vi "PAtestingworks.vi"() -> ()   [LabVIEW 2014]
uses:
  <vilib>/vision/NI_Vision_Development_Module.lvlib
  <instrlib>/KD Scientific 2XX Series/KD Scientific 2XX Series.lvlib
panel:
  in  "Number of Cycles":i32
  in  "Min Pressure":dbl
  in  "Max Pressure":dbl
  out "Status":T1
  in  "stop 2":bool
  out "Delivered Volume":dbl
  out "Units":string
  in  "Baud Rate (9600)":u32(ring)=9600 items=["300"=300, "1200"=1200, "2400"=2400, "4800"=4800, "9600"=9600]
  in  "Withdrawal Settings":T2={"Flow Rate (5)"=5.0, "Volume (10)"=10.0, "Volume Units (ml)"=enum."milliliters (ml)", "Rate Units (ml/min.)"=enum."milliliters per minute (ml/min.)"} {"Volume (10)" format="%#.3g"}
  in  "Diameter (8.75 mm)":dbl=8.75
  in  "Infusion Settings":T2={"Flow Rate (5)"=5.0, "Volume (10)"=10.0, "Volume Units (ml)"=enum."milliliters (ml)", "Rate Units (ml/min.)"=enum."milliliters per minute (ml/min.)"}
  in  "Address (0)":i32 format="%0.0f"
  in  "error in (no error)":errorcluster
  in  "VISA resource name":refnum<visa-resource-name>="COM1"
  in  "stop":bool
  out "Image":T3(plugin-control)
  out "Particle Measurements (Pixels) (Particle Analysis 1)":dbl[][](array[numeric]) format="%.2f"
  out "subarray":dbl[](array[numeric])
  out "The diameter":dbl[](array[numeric])
  in  "stop (F)":bool
  out "Data from Transducer":dynamicdata(graph) caption="Voltage from Transducer V"
  out "Voltage from pressure transducer":dbl[](array[numeric])
  out "Pressure mm Hg":dbl[](graph)
  in  "Calibration factor":dbl[](array[numeric])
  in  "Zero Error":dbl[](array[numeric])
  out "pressure mm Hg":dbl[](array[numeric])
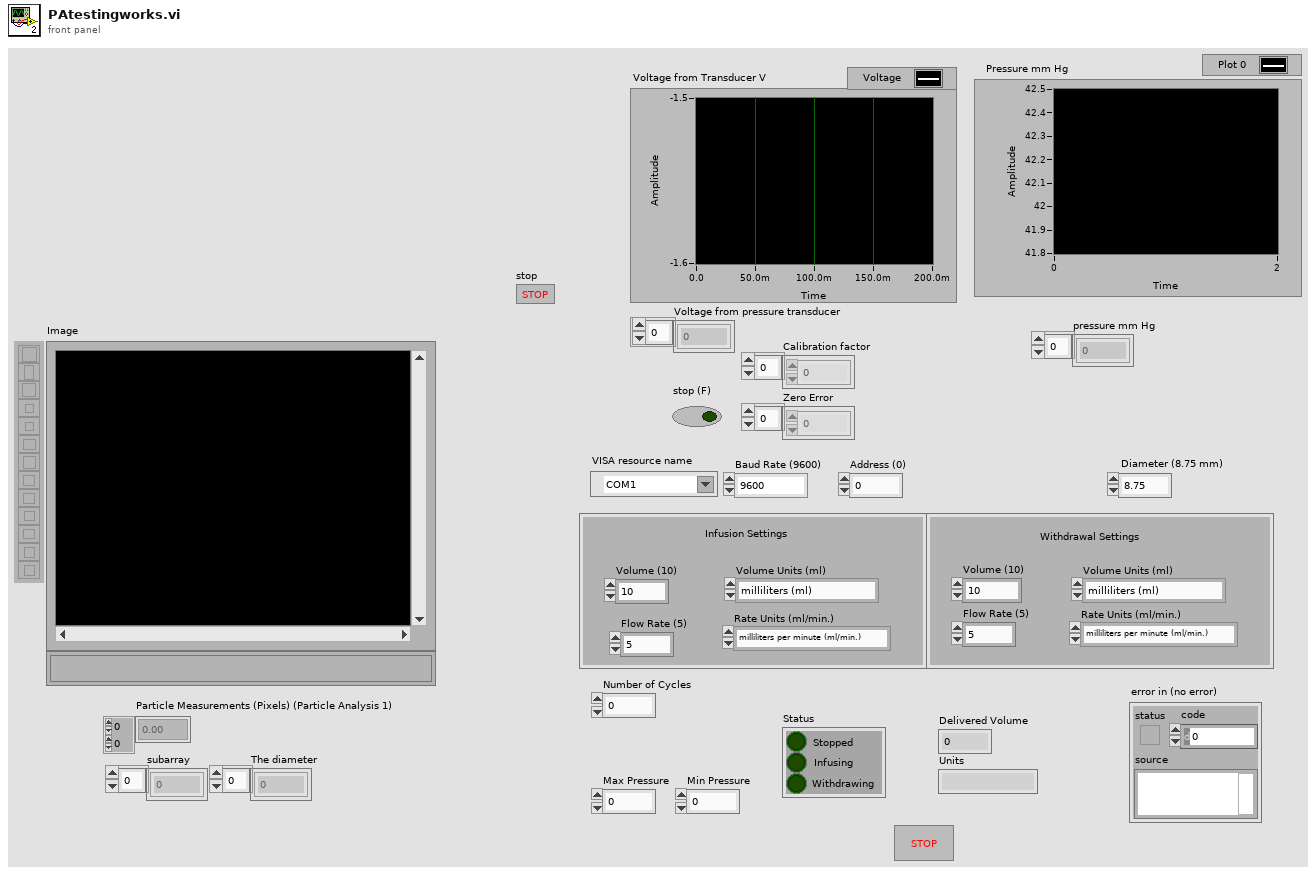
[diagram p1: front panel]
types:
  T1 = cluster{"Stopped":bool, "Infusing":bool, "Withdrawing":bool}
  T2 = cluster{"Flow Rate (5)":dbl, "Volume (10)":dbl, "Volume Units (ml)":enum16{"milliliters (ml)", "microliters (ul)"}, "Rate Units (ml/min.)":enum16{"milliliters per minute (ml/min.)", "milliliters per hour (ml/hr.)", "microliters per minute (ul/min.)", "microliters per hour (ul/hr.)"}}
  T3 = typedef "IMAQ Image.ctl" = refnum<image>
  T4 = typedef "Board Id" = u8
  T5 = typedef "ROI Descriptor" = cluster{"Global Rectangle":i32[], "Contours":cluster{"ID":enum32{"External", "Internal"}, "Type":u32, "Coordinates":i32[]}[]}
  T6 = enum16{"milliliters per minute (ml/min.)", "milliliters per hour (ml/hr.)", "microliters per minute (ul/min.)", "microliters per hour (ul/hr.)"}
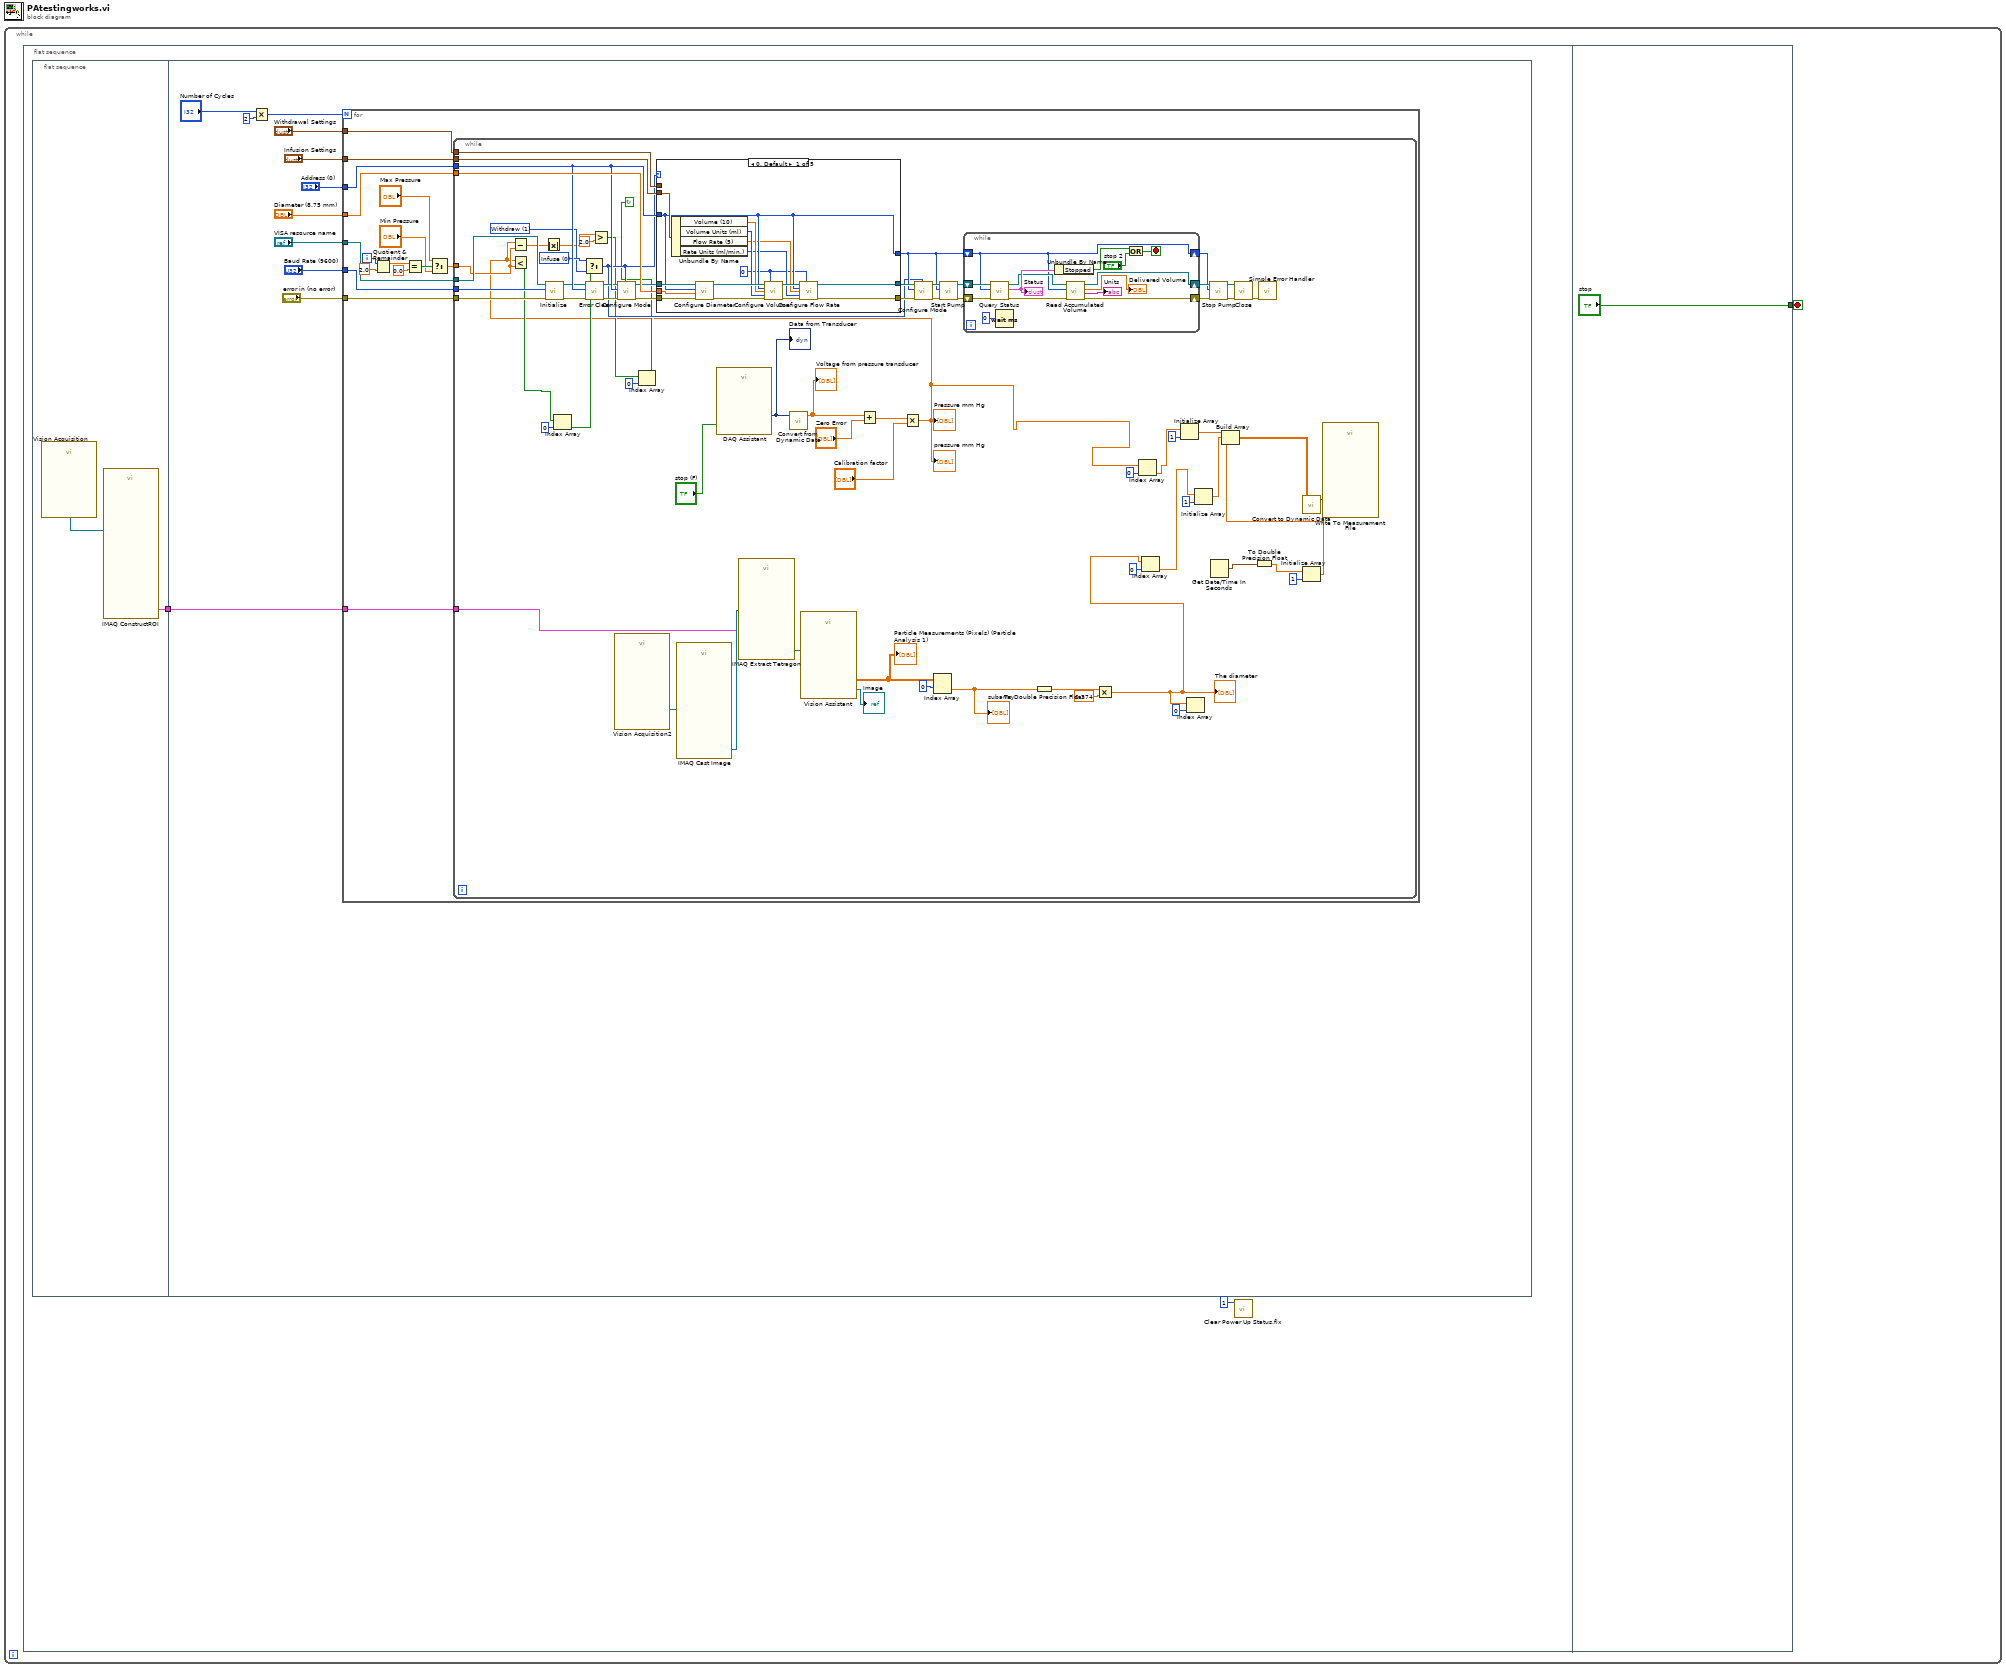
[diagram p0: block diagram]
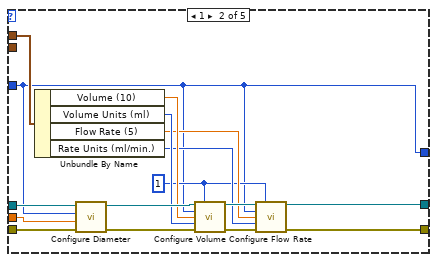
[diagram p2: hidden frame]
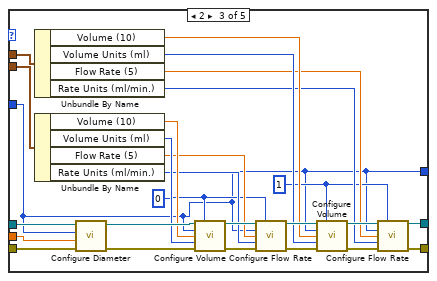
[diagram p3: hidden frame]
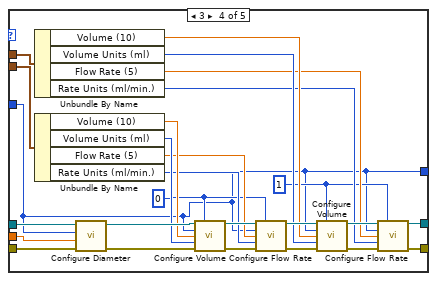
[diagram p4: hidden frame]
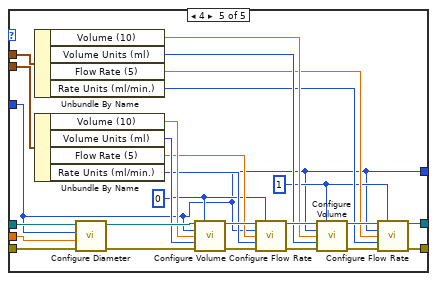
[diagram p5: hidden frame]
diagram:
  n1 = while {
    stop <- w1 stop-if-true
    n2 = flat-sequence {
      tunnel: ["stop"] -> w1
      frame #0 {
        n3 = flat-sequence {
          tunnel: [w4] -> w3
          tunnel: w3 -> [w7]
          frame #0 {
            n4 = call "Vision Acquisition"() -> ("Image Out"=w5:T3)  [unwired: 26 in, 1 out]
            n5 = call "IMAQ ConstructROI"("Image"=w5) -> ("ROI Descriptor Out"=w4:T5)  [unwired: 7 in, 3 out]
          }
          frame #1 {
            n6 = Multiply(x="Number of Cycles", y=2) -> (x*y=w6:i32)
            n7 = for {
              N: w6 -> [_]
              tunnel: "VISA resource name" -> [w32]
              tunnel: "error in (no error)" -> [w31]
              tunnel: "Infusion Settings" -> [w30]
              tunnel: "Withdrawal Settings" -> [w29]
              tunnel: "Diameter (8.75 mm)" -> [w28]
              tunnel: "Baud Rate (9600)" -> [w27]
              tunnel: "Address (0)" -> [w26]
              tunnel: w7 -> [w17]
              i -> [w24]
              n8 = Quotient & Remainder(x=w24, y=2.0) -> (x-y*floor(x/y)=w22:dbl)  [unwired: 1 out]
              n9 = Equal?(x=w22, y=0.0) -> (x = y?=w21:bool)
              n10 = Select(t="Max Pressure", s=w21, f="Min Pressure") -> (s? t:f=w18:dbl)
              n11 = while {
                tunnel: w32 -> [w104]
                tunnel: w31 -> [w103]
                tunnel: w30 -> [w102]
                tunnel: w29 -> [w101]
                tunnel: w28 -> [w100]
                tunnel: w27 -> [w99]
                tunnel: w26 -> [w98]
                tunnel: w18 -> [w75]
                tunnel: w17 -> [w49]
                stop <- w60 continue-if-true
                w77 = u16 1 items=["Withdraw"=1]
                w78 = u16 0 items=["Infuse"] ("Mode (infuse)")
                n12 = call <instrlib>:"Initialize.vi"("error in (no error)"=w103, "Baud Rate (9600)"=w99, "VISA resource name"=w104) -> ("error out"=w80:errorcluster, "VISA resource name out"=w79:refnum<visa-resource-name>)  [unwired: 7 in]
                n13 = call <instrlib>:"Error Clear.vi"("error in (no error)"=w80, "Address (0)"=w98, "VISA resource name"=w79) -> ("error out"=w81:errorcluster, "VISA resource name out"=w82:refnum<visa-resource-name>)  [unwired: 6 in, 1 out]
                n14 = call "Vision Acquisition2"() -> ("Image Out"=w59:T3)  [unwired: 25 in, 2 out]
                n15 = call "IMAQ Cast Image"("Image Src"=w59) -> ("Image Dst Out"=w52:T3)  [unwired: 9 in, 1 out]
                n16 = call "DAQ Assistant"("stop (T)"="stop (F)") -> ("data"=w66:dynamicdata)  [unwired: 16 in, 2 out]
                "Data from Transducer" <- w66
                n17 = call-poly "IMAQ Extract Tetragon"("ROI Descriptor"=w49, "Image Src"=w52) -> ("Image Dst Out"=w51:T3)  [unwired: 8 in, 1 out]
                n18 = call "Convert from Dynamic Data"("Dynamic Data Type"=w66) -> ("Array"=w69:dbl[])  [unwired: 3 in]
                "Voltage from pressure transducer" <- w69
                n19 = call "Vision Assistant"("Image In"=w51) -> ("Image Out"=→"Image":T3, "Particle Measurements (Pixels) (Particle Analysis 1)"=w53:dbl[][])  [unwired: 23 in, 2 out]
                "Particle Measurements (Pixels) (Particle Analysis 1)" <- w53
                n20 = Add(x=w69, y="Zero Error") -> (x+y=w67:dbl[])
                n21 = Multiply(x=w67, y="Calibration factor") -> (x*y=w45:dbl[])
                "Pressure mm Hg" <- w45
                "pressure mm Hg" <- w45
                n22 = Subtract(x=w45, y=w75) -> (x-y=w74:dbl[])
                n23 = Less?(x=w45, y=w75) -> (x < y?=w65:bool[])
                n24 = Absolute Value(x=w74) -> (abs(x)=w73:dbl[])
                n25 = Index Array(array=w65, index=0) -> (element=w63:bool)
                n26 = Select(t=w78, s=w63, f=w77) -> (s? t:f=w76:u16)
                n27 = Greater?(x=w73, y=2.0) -> (0:w62:bool[])
                n28 = call <instrlib>:"Configure Mode.vi"("Mode (infuse)"=w76, "error in (no error)"=w81, "Address (0)"=w98, "VISA resource name"=w82) -> ("error out"=w84:errorcluster, "VISA resource name out"=w83:refnum<visa-resource-name>)  [unwired: 6 in]
                n29 = Index Array(array=w62, index=0) -> (element=w60:bool)
                n30 = case shown="0, Default" w76 {
                  tunnel: w102 -> [w114 _ w162 w188 w214]
                  tunnel: w101 -> [_ w136 w161 w187 w213]
                  tunnel: w83 -> [w120 w135 w160 w186 w212]
                  tunnel: w84 -> [w119 w131 w159 w185 w211]
                  tunnel: w100 -> [w113 w127 w142 w168 w194]
                  tunnel: [w112 w121 w137 w163 w189] -> w85
                  tunnel: w98 -> [w112 w121 w137 w163 w189]
                  tunnel: [w107 w132 w139 w165 w191] -> w89
                  tunnel: [w106 w128 w138 w164 w190] -> w88
                  frame 0, Default {
                    w105 = 0
                    n31 = Unbundle By Name(w114) -> ("Volume (10)"=w111:dbl, "Volume Units (ml)"=w110:enum16{"milliliters (ml)", "microliters (ul)"}, "Flow Rate (5)"=w109:dbl, "Rate Units (ml/min.)"=w108:T6)
                    n32 = call <instrlib>:"Configure Diameter.vi"("error in (no error)"=w119, "Diameter (8.75 mm)"=w113, "Address (0)"=w112, "VISA resource name"=w120) -> ("error out"=w117:errorcluster, "VISA resource name out"=w118:refnum<visa-resource-name>)  [unwired: 6 in]
                    n33 = call <instrlib>:"Configure Volume.vi"("VISA resource name"=w118, "Mode (infuse)"=w105, "Address (0)"=w112, "Volume (100)"=w111, "Units (0: milliliters)"=w110, "error in (no error)"=w117) -> ("VISA resource name out"=w116:refnum<visa-resource-name>, "error out"=w115:errorcluster)  [unwired: 8 in]
                    n34 = call <instrlib>:"Configure Flow Rate.vi"("VISA resource name"=w116, "Mode (infuse)"=w105, "Address (0)"=w112, "Flow Rate (5)"=w109, "Units (0: milliliters per minute)"=w108, "error in (no error)"=w115) -> ("VISA resource name out"=w107:refnum<visa-resource-name>, "error out"=w106:errorcluster)  [unwired: 8 in]
                  }
                  frame 1 {
                    w122 = 1
                    n35 = Unbundle By Name(w136) -> ("Volume (10)"=w126:dbl, "Volume Units (ml)"=w125:enum16{"milliliters (ml)", "microliters (ul)"}, "Flow Rate (5)"=w124:dbl, "Rate Units (ml/min.)"=w123:T6)
                    n36 = call <instrlib>:"Configure Diameter.vi"("error in (no error)"=w131, "Diameter (8.75 mm)"=w127, "Address (0)"=w121, "VISA resource name"=w135) -> ("error out"=w130:errorcluster, "VISA resource name out"=w134:refnum<visa-resource-name>)  [unwired: 6 in]
                    n37 = call <instrlib>:"Configure Volume.vi"("VISA resource name"=w134, "Mode (infuse)"=w122, "Address (0)"=w121, "Volume (100)"=w126, "Units (0: milliliters)"=w125, "error in (no error)"=w130) -> ("VISA resource name out"=w133:refnum<visa-resource-name>, "error out"=w129:errorcluster)  [unwired: 8 in]
                    n38 = call <instrlib>:"Configure Flow Rate.vi"("VISA resource name"=w133, "Mode (infuse)"=w122, "Address (0)"=w121, "Flow Rate (5)"=w124, "Units (0: milliliters per minute)"=w123, "error in (no error)"=w129) -> ("VISA resource name out"=w132:refnum<visa-resource-name>, "error out"=w128:errorcluster)  [unwired: 8 in]
                  }
                  frame 2 {
                    w140 = 1
                    w141 = 0
                    n39 = Unbundle By Name(w161) -> ("Volume (10)"=w146:dbl, "Volume Units (ml)"=w145:enum16{"milliliters (ml)", "microliters (ul)"}, "Flow Rate (5)"=w144:dbl, "Rate Units (ml/min.)"=w143:T6)
                    n40 = Unbundle By Name(w162) -> ("Volume (10)"=w150:dbl, "Volume Units (ml)"=w149:enum16{"milliliters (ml)", "microliters (ul)"}, "Flow Rate (5)"=w148:dbl, "Rate Units (ml/min.)"=w147:T6)
                    n41 = call <instrlib>:"Configure Diameter.vi"("error in (no error)"=w159, "Diameter (8.75 mm)"=w142, "Address (0)"=w137, "VISA resource name"=w160) -> ("error out"=w154:errorcluster, "VISA resource name out"=w158:refnum<visa-resource-name>)  [unwired: 6 in]
                    n42 = call <instrlib>:"Configure Volume.vi"("VISA resource name"=w158, "Mode (infuse)"=w141, "Address (0)"=w137, "Volume (100)"=w150, "Units (0: milliliters)"=w149, "error in (no error)"=w154) -> ("VISA resource name out"=w157:refnum<visa-resource-name>, "error out"=w153:errorcluster)  [unwired: 8 in]
                    n43 = call <instrlib>:"Configure Flow Rate.vi"("VISA resource name"=w157, "Mode (infuse)"=w141, "Address (0)"=w137, "Flow Rate (5)"=w148, "Units (0: milliliters per minute)"=w147, "error in (no error)"=w153) -> ("VISA resource name out"=w156:refnum<visa-resource-name>, "error out"=w152:errorcluster)  [unwired: 8 in]
                    n44 = call <instrlib>:"Configure Volume.vi"("VISA resource name"=w156, "Mode (infuse)"=w140, "Address (0)"=w137, "Volume (100)"=w146, "Units (0: milliliters)"=w145, "error in (no error)"=w152) -> ("VISA resource name out"=w155:refnum<visa-resource-name>, "error out"=w151:errorcluster)  [unwired: 8 in]
                    n45 = call <instrlib>:"Configure Flow Rate.vi"("VISA resource name"=w155, "Mode (infuse)"=w140, "Address (0)"=w137, "Flow Rate (5)"=w144, "Units (0: milliliters per minute)"=w143, "error in (no error)"=w151) -> ("VISA resource name out"=w139:refnum<visa-resource-name>, "error out"=w138:errorcluster)  [unwired: 8 in]
                  }
                  frame 3 {
                    w166 = 1
                    w167 = 0
                    n46 = Unbundle By Name(w187) -> ("Volume (10)"=w172:dbl, "Volume Units (ml)"=w171:enum16{"milliliters (ml)", "microliters (ul)"}, "Flow Rate (5)"=w170:dbl, "Rate Units (ml/min.)"=w169:T6)
                    n47 = Unbundle By Name(w188) -> ("Volume (10)"=w176:dbl, "Volume Units (ml)"=w175:enum16{"milliliters (ml)", "microliters (ul)"}, "Flow Rate (5)"=w174:dbl, "Rate Units (ml/min.)"=w173:T6)
                    n48 = call <instrlib>:"Configure Diameter.vi"("error in (no error)"=w185, "Diameter (8.75 mm)"=w168, "Address (0)"=w163, "VISA resource name"=w186) -> ("error out"=w180:errorcluster, "VISA resource name out"=w184:refnum<visa-resource-name>)  [unwired: 6 in]
                    n49 = call <instrlib>:"Configure Volume.vi"("VISA resource name"=w184, "Mode (infuse)"=w167, "Address (0)"=w163, "Volume (100)"=w176, "Units (0: milliliters)"=w175, "error in (no error)"=w180) -> ("VISA resource name out"=w183:refnum<visa-resource-name>, "error out"=w179:errorcluster)  [unwired: 8 in]
                    n50 = call <instrlib>:"Configure Flow Rate.vi"("VISA resource name"=w183, "Mode (infuse)"=w167, "Address (0)"=w163, "Flow Rate (5)"=w174, "Units (0: milliliters per minute)"=w173, "error in (no error)"=w179) -> ("VISA resource name out"=w182:refnum<visa-resource-name>, "error out"=w178:errorcluster)  [unwired: 8 in]
                    n51 = call <instrlib>:"Configure Volume.vi"("VISA resource name"=w182, "Mode (infuse)"=w166, "Address (0)"=w163, "Volume (100)"=w172, "Units (0: milliliters)"=w171, "error in (no error)"=w178) -> ("VISA resource name out"=w181:refnum<visa-resource-name>, "error out"=w177:errorcluster)  [unwired: 8 in]
                    n52 = call <instrlib>:"Configure Flow Rate.vi"("VISA resource name"=w181, "Mode (infuse)"=w166, "Address (0)"=w163, "Flow Rate (5)"=w170, "Units (0: milliliters per minute)"=w169, "error in (no error)"=w177) -> ("VISA resource name out"=w165:refnum<visa-resource-name>, "error out"=w164:errorcluster)  [unwired: 8 in]
                  }
                  frame 4 {
                    w192 = 1
                    w193 = 0
                    n53 = Unbundle By Name(w213) -> ("Volume (10)"=w198:dbl, "Volume Units (ml)"=w197:enum16{"milliliters (ml)", "microliters (ul)"}, "Flow Rate (5)"=w196:dbl, "Rate Units (ml/min.)"=w195:T6)
                    n54 = Unbundle By Name(w214) -> ("Volume (10)"=w202:dbl, "Volume Units (ml)"=w201:enum16{"milliliters (ml)", "microliters (ul)"}, "Flow Rate (5)"=w200:dbl, "Rate Units (ml/min.)"=w199:T6)
                    n55 = call <instrlib>:"Configure Diameter.vi"("error in (no error)"=w211, "Diameter (8.75 mm)"=w194, "Address (0)"=w189, "VISA resource name"=w212) -> ("error out"=w206:errorcluster, "VISA resource name out"=w210:refnum<visa-resource-name>)  [unwired: 6 in]
                    n56 = call <instrlib>:"Configure Volume.vi"("VISA resource name"=w210, "Mode (infuse)"=w193, "Address (0)"=w189, "Volume (100)"=w202, "Units (0: milliliters)"=w201, "error in (no error)"=w206) -> ("VISA resource name out"=w209:refnum<visa-resource-name>, "error out"=w205:errorcluster)  [unwired: 8 in]
                    n57 = call <instrlib>:"Configure Flow Rate.vi"("VISA resource name"=w209, "Mode (infuse)"=w193, "Address (0)"=w189, "Flow Rate (5)"=w200, "Units (0: milliliters per minute)"=w199, "error in (no error)"=w205) -> ("VISA resource name out"=w208:refnum<visa-resource-name>, "error out"=w204:errorcluster)  [unwired: 8 in]
                    n58 = call <instrlib>:"Configure Volume.vi"("VISA resource name"=w208, "Mode (infuse)"=w192, "Address (0)"=w189, "Volume (100)"=w198, "Units (0: milliliters)"=w197, "error in (no error)"=w204) -> ("VISA resource name out"=w207:refnum<visa-resource-name>, "error out"=w203:errorcluster)  [unwired: 8 in]
                    n59 = call <instrlib>:"Configure Flow Rate.vi"("VISA resource name"=w207, "Mode (infuse)"=w192, "Address (0)"=w189, "Flow Rate (5)"=w196, "Units (0: milliliters per minute)"=w195, "error in (no error)"=w203) -> ("VISA resource name out"=w191:refnum<visa-resource-name>, "error out"=w190:errorcluster)  [unwired: 8 in]
                  }
                }
                n60 = call <instrlib>:"Configure Mode.vi"("Mode (infuse)"=w76, "error in (no error)"=w88, "Address (0)"=w85, "VISA resource name"=w89) -> ("error out"=w86:errorcluster, "VISA resource name out"=w87:refnum<visa-resource-name>)  [unwired: 6 in]
                n61 = Index Array(array=w53, index (row)=0) -> (element=w55:dbl[])  [unwired: 1 in]
                "subarray" <- w55
                n62 = call <instrlib>:"Start Pump.vi"("error in (no error)"=w86, "Address (0)"=w85, "VISA resource name"=w87) -> ("error out"=w96:errorcluster, "VISA resource name out"=w97:refnum<visa-resource-name>)  [unwired: 7 in]
                n63 = while {
                  shift-right: [w217] -> w93
                  shift-left: w85 -> [w217]
                  shift-right: [w219] -> w95
                  shift-left: w97 -> [w225]
                  shift-right: [w218] -> w94
                  shift-left: w96 -> [w226]
                  stop <- w223 stop-if-true
                  n64 = call <instrlib>:"Query Status.vi"("error in (no error)"=w226, "Address (0)"=w217, "VISA resource name"=w225) -> ("error out"=w228:errorcluster, "Status"=w224:T1, "VISA resource name out"=w220:refnum<visa-resource-name>)  [unwired: 6 in]
                  "Status" <- w224
                  n65 = Wait (ms)(milliseconds to wait=u32 0) -> ()  [unwired: 1 out]
                  n66 = Unbundle By Name(w224) -> ("Stopped"=w222:bool)
                  n67 = call <instrlib>:"Read Accumulated Volume.vi"("error in (no error)"=w228, "Address (0)"=w217, "VISA resource name"=w220) -> ("error out"=w218:errorcluster, "Units"=→"Units":string, "Delivered Volume"=→"Delivered Volume":dbl, "VISA resource name out"=w219:refnum<visa-resource-name>)  [unwired: 5 in]
                  n68 = Or(x=w222, y="stop 2") -> (x .or. y?=w223:bool)
                }
                n69 = To Double Precision Float(number=w55) -> (double precision float=w56:dbl[])
                n70 = Multiply(x=w56, y=0.374) -> (x*y=w46:dbl[])
                "The diameter" <- w46
                n71 = Index Array(array=w45, index=0) -> (element=w42:dbl)
                n72 = Index Array(array=w46, index=0) -> (element=w41:dbl)
                n73 = Initialize Array(w42, 1 ("dimension size")) -> (w40:dbl[])
                n74 = Index Array(array=w46, index=0) -> ()  [unwired: 1 out]
                n75 = Initialize Array(w41, 1 ("dimension size")) -> (w39:dbl[])
                n76 = call <instrlib>:"Stop Pump.vi"("error in (no error)"=w94, "Address (0)"=w93, "VISA resource name"=w95) -> ("error out"=w91:errorcluster, "VISA resource name out"=w90:refnum<visa-resource-name>)  [unwired: 7 in]
                n77 = Get Date/Time In Seconds() -> (seconds since 1Jan1904=w38:timestamp)
                n78 = call <instrlib>:"Close.vi"("error in (no error)"=w91, "VISA resource name"=w90) -> ("error out"=w92:errorcluster)  [unwired: 9 in]
                n79 = To Double Precision Float(number=w38) -> (double precision float=w37:dbl)
                n80 = call <vilib>:"Simple Error Handler.vi"("error in (no error)"=w92) -> ()  [unwired: 4 in, 5 out]
                n81 = Initialize Array(w37, 1 ("dimension size")) -> (w35:dbl[])
                n82 = Build Array(w40, w39, w35) -> (w34:dbl[][])
                n83 = call "Convert to Dynamic Data"("2D Array"=w34) -> ("Dynamic Data Type"=w33:dynamicdata)  [unwired: 3 in]
                n84 = call "Write To Measurement File"("Signals"=w33) -> ()  [unwired: 16 in, 3 out]
              }
            }
          }
        }
        n85 = call <vilib>:"Clear Power Up Status.flx"("Board ID"=T4 1) -> ()  [unwired: 6 in, 2 out]
      }
      frame #1 {
      }
    }
  }
